vi "Secure WebSocket Server Test with dotNET.vi"() -> ()   [LabVIEW 2013]
uses:
  dotNET SSL Socket/dotNET SSL Listener/dotNET Listener.lvclass
  dotNET SSL Socket/dotNET SSL Server/dotNET SSL Server.lvclass/dotNET SSL Server.ctl
  dotNET SSL Socket/dotNET SSL Server/dotNET SSL Server.lvclass
  <vilib>/MediaMongrels Ltd/WebSockets/WebSockets/WebSocket Server/WebSocket Server.lvclass
  <vilib>/MediaMongrels Ltd/WebSockets/WebSockets/WebSocket/WebSocket.lvclass/WebSocket.ctl
  dotNET SSL Socket/dotNET SSL Server/Write PFX Certificate.vi
  dotNET SSL Socket/dotNET SSL Server/Write PFX Password.vi
  <vilib>/MediaMongrels Ltd/WebSockets/WebSockets/WebSocket/Read Return Headers.vi
panel:
  out "error out":errorcluster
  out "RX Data":string
  out "Return Headers":variant
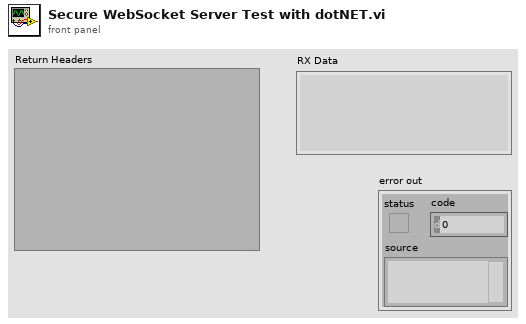
[diagram p1: front panel]
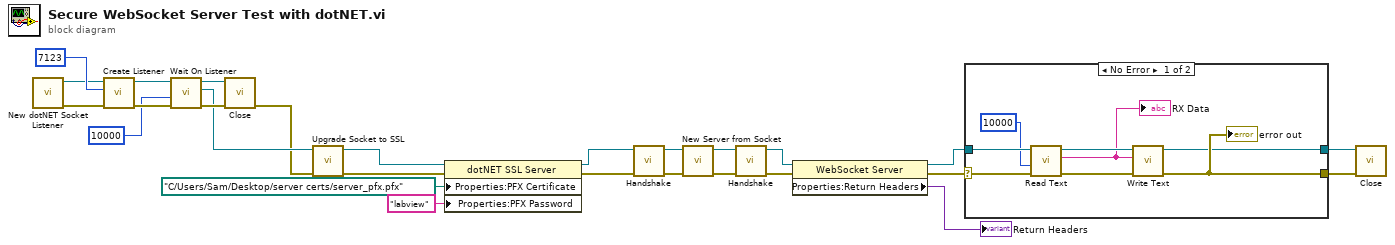
[diagram p0: block diagram]
diagram:
  n1 = call "New dotNET Socket Listener.vi"() -> ("error out"=w2:errorcluster, "dotNET Listener out"=w1:refnum<class "dotNET Listener.lvclass">)  [unwired: 10 in]
  n2 = call-dynamic "Create Listener.vi"("error in (no error)"=w2, "Port"=u16 7123 ("port"), "dotNET Listener in"=w1) -> ("error out"=w18:errorcluster, "dotNET Listener out"=w15:refnum<class "dotNET Listener.lvclass">)  [unwired: 7 in]
  n3 = call-dynamic "Wait On Listener.vi"("error in (no error)"=w18, "timeout ms (5000)"=10000, "dotNET Listener in"=w15) -> ("error out"=w17:errorcluster, "Socket out"=w11:refnum<class "Socket.lvclass">, "dotNET Listener out"=w16:refnum<class "dotNET Listener.lvclass">)  [unwired: 6 in]
  n4 = call-dynamic "Close.vi"("error in (no error)"=w17, "dotNET Listener in"=w16) -> ("error out"=w10:errorcluster)  [unwired: 9 in]
  n5 = call "Upgrade Socket to SSL.vi"("error in (no error)"=w10, "Socket in"=w11) -> ("error out"=w14:errorcluster, "dotNET SSL Socket out"=w7:refnum<class "dotNET SSL Server.lvclass">)  [unwired: 8 in]
  n6 = property class="dotNET SSL Server"(reference=w7, error in=w14, "Properties:PFX Certificate"=path "C:/Users/Sam/Desktop/server certs/server_pfx.pfx" ("PFX Certificate"), "Properties:PFX Password"="labview" ("PFX Password")) -> (reference out=w6:refnum<class "dotNET SSL Server.lvclass">, error out=w8:errorcluster)
  n7 = call-dynamic "Handshake.vi"("error in (no error)"=w8, "dotNET SSL Socket in"=w6) -> ("error out"=w12:errorcluster, "dotNET SSL Socket out"=w13:refnum<class "dotNET SSL Server.lvclass">)  [unwired: 8 in]
  n8 = call <vilib>:"New Server from Socket.vi"("error in (no error)"=w12, "Socket"=w13) -> ("error out"=w27:errorcluster, "WebSocket Server out"=w26:refnum<class "WebSocket Server.lvclass">)  [unwired: 8 in]
  n9 = call-dynamic "Handshake.vi"("error in (no error)"=w27, "WebSocket Connection in"=w26) -> ("error out"=w25:errorcluster, "WebSocket Connection out"=w24:refnum<class "WebSocket Server.lvclass">)  [unwired: 8 in]
  n10 = property class="WebSocket Server"(reference=w24, error in=w25) -> (reference out=w22:refnum<class "WebSocket Server.lvclass">, error out=w19:errorcluster, "Properties:Return Headers"=→"Return Headers":variant)
  n11 = case shown="No Error" w19 {
    selector: w19 -> [w32 w36]
    tunnel: w22 -> [w35 w37]
    tunnel: [w34 w36] -> w21
    tunnel: [w33 w37] -> w20
    frame No Error {
      n12 = call-dynamic "Read Text.vi"("error in (no error)"=w32, "timeout ms (5000)"=10000, "WebSocket in"=w35) -> ("error out"=w30:errorcluster, "Data"=w28:string, "WebSocket out"=w29:refnum<class "WebSocket Server.lvclass">)  [unwired: 6 in]
      "RX Data" <- w28
      n13 = call-dynamic "Write Text.vi"("error in (no error)"=w30, "String Data"=w28, "WebSocket in"=w29) -> ("error out"=w34:errorcluster, "WebSocket out"=w33:refnum<class "WebSocket Server.lvclass">)  [unwired: 7 in]
      "error out" <- w34
    }
    frame Error {
    }
  }
  n14 = call-dynamic "Close.vi"("error in (no error)"=w21, "WebSocket in"=w20) -> ()  [unwired: 9 in, 1 out]
